vi "morseSignReader.vi"(10 "current morse sign":string, 11 "Enum":T1(ring)) -> (3 "f":string)   [LabVIEW 2017]
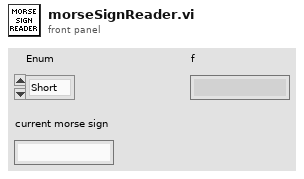
[diagram p1: front panel]
types:
  T1 = enum16{"Short", "Long", "No update", "Evaluate and Null String"}
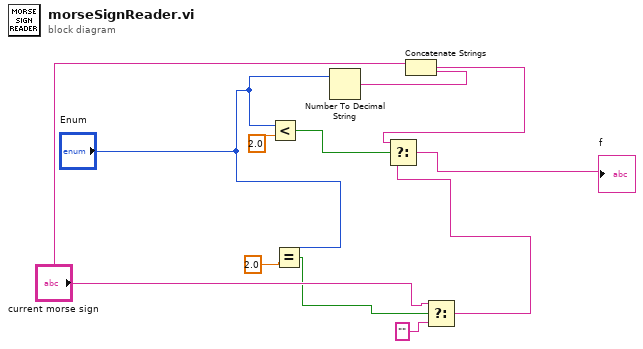
[diagram p0: block diagram]
diagram:
  n1 = Less?(x="Enum", y=2.0) -> (x < y?=w1:bool)
  n2 = Equal?(x="Enum", y=2.0) -> (x = y?=w7:bool)
  n3 = Number To Decimal String(number="Enum") -> (decimal integer string=w5:string)  [unwired: 1 in]
  n4 = Concatenate Strings("current morse sign", w5) -> (w4:string)
  n5 = Select(t="current morse sign", s=w7, f="") -> (s? t:f=w8:string)
  n6 = Select(t=w4, s=w1, f=w8) -> (s? t:f=→"f":string)
